vi "DisplaySettings from INI Section.vi"(8 "error in (no error)":errorcluster, 11 "refnum in":T2) -> (0 "error out":errorcluster, 2 "Display settings":T1={"Min. Thresh."=0.0, "X"=0.0, "Y"=0.0, "ShowLineout"=FALSE, "ScaleParts"=10, "ShowLegende"=FALSE, "Target Cross"=FALSE, "Centroid Cross"=FALSE, "Target color"=16777226, "Centroid color"=16711680, "calibr. mm/px"=0.0}, 3 "refnum out":T2)   [LabVIEW 2020, in "POLARIS IMAQ Display.xctl"]
uses:
  POLARIS IMAQ Display.xctl
  <vilib>/Utility/config.llb/Config Data RefNum.ctl
  DisplaySettings.ctl
  <vilib>/Utility/config.llb/Read Key (Double).vi
  <vilib>/Utility/config.llb/NI_LVConfig.lvlib
panel:
  in  "Display settings 2":T1={"Min. Thresh."=0.0, "X"=0.0, "Y"=0.0, "ShowLineout"=FALSE, "ScaleParts"=10, "ShowLegende"=FALSE, "Target Cross"=TRUE, "Centroid Cross"=TRUE, "Target color"=16777226, "Centroid color"=16711680, "calibr. mm/px"=0.0}
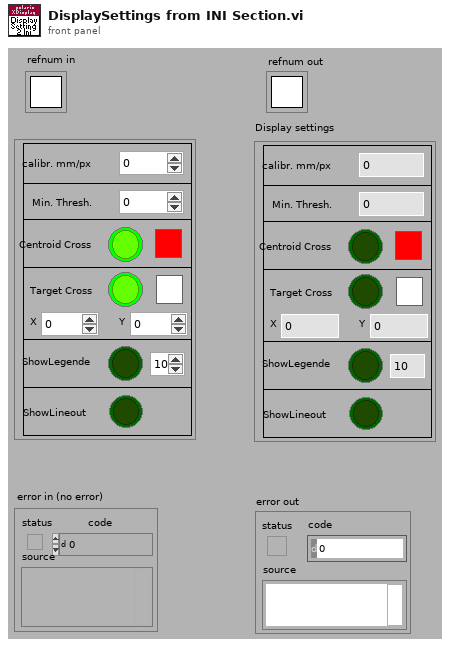
[diagram p1: front panel]
types:
  T1 = typedef "POLARIS IMAQ Display.xctl/DisplaySettings.ctl" = cluster{"Min. Thresh.":sgl, "X":dbl, "Y":dbl, "ShowLineout":bool, "ScaleParts":i32, "ShowLegende":bool, "Target Cross":bool, "Centroid Cross":bool, "Target color":u32, "Centroid color":u32, "calibr. mm/px":sgl}
  T2 = typedef "NI_LVConfig.lvlib/Config Data RefNum.ctl" = refnum<k1>
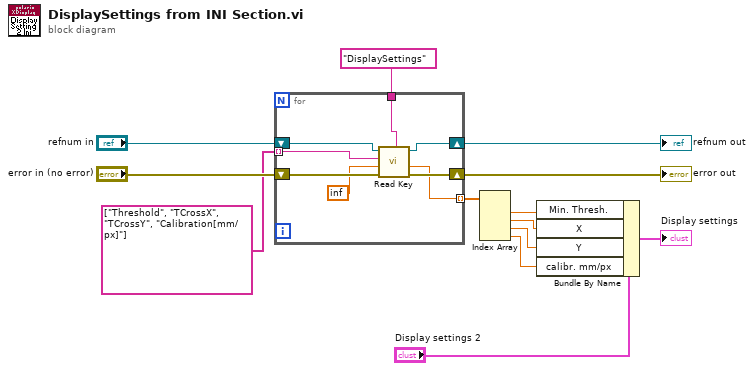
[diagram p0: block diagram]
diagram:
  n1 = for {
    tunnel: "DisplaySettings" ("section") -> [w20]
    shift-right: [w15] -> w9
    shift-left: "error in (no error)" -> [w18]
    tunnel: string[] ["Threshold", "TCrossX", "TCrossY", "Calibration[mm/px]"] -> [w19] mode=indexing
    shift-right: [w16] -> w12
    shift-left: "refnum in" -> [w21]
    tunnel: [w14] -> w6 mode=indexing
    n2 = call-poly <vilib>:"Read Key.vi"("section"=w20, "error in (no error)"=w18, "default value"=inf, "key"=w19, "refnum"=w21) -> ("error out"=w15:errorcluster, "value"=w14:dbl, "refnum out"=w16:T2)  [unwired: 3 in, 1 out]
  }
  "refnum out" <- w12
  "error out" <- w9
  n3 = Index Array(array=w6) -> (element #1=w5:dbl, element #2=w4:dbl, element #3=w3:dbl, element #4=w2:dbl)  [unwired: 4 in]
  n4 = Bundle By Name(cluster="Display settings 2", "Min. Thresh."=w5, "X"=w4, "Y"=w3, "calibr. mm/px"=w2) -> (→"Display settings":T1)
